vi "DecodeTopicSubscribeReply.vi"(3 "Topic Reply":string="POST / HTTP/1.1\r\nUser-Agent: XMLRPC++ 0.7\r\nHost: 192.168.1.111:5000\r\nContent-Type: text/xml\r\nContent-length: 330\r\n\r\n<?xml version=\"1.0\"?>\r\n<methodCall><methodName>requestTopic</methodName>\r\n<params><param><value>/realtime_loop</value></param><param><value>/robot/head/command_head_nod</value></param><param><value><array><data><value><array><data><value>TCPROS</value></data></array></value></data></array></value></param></params></methodCall>\r\n") -> (0 "error out":errorcluster, 1 "Reply":T1(array[cluster]))   [LabVIEW 2012]
panel:
  in  "error in (no error)":errorcluster
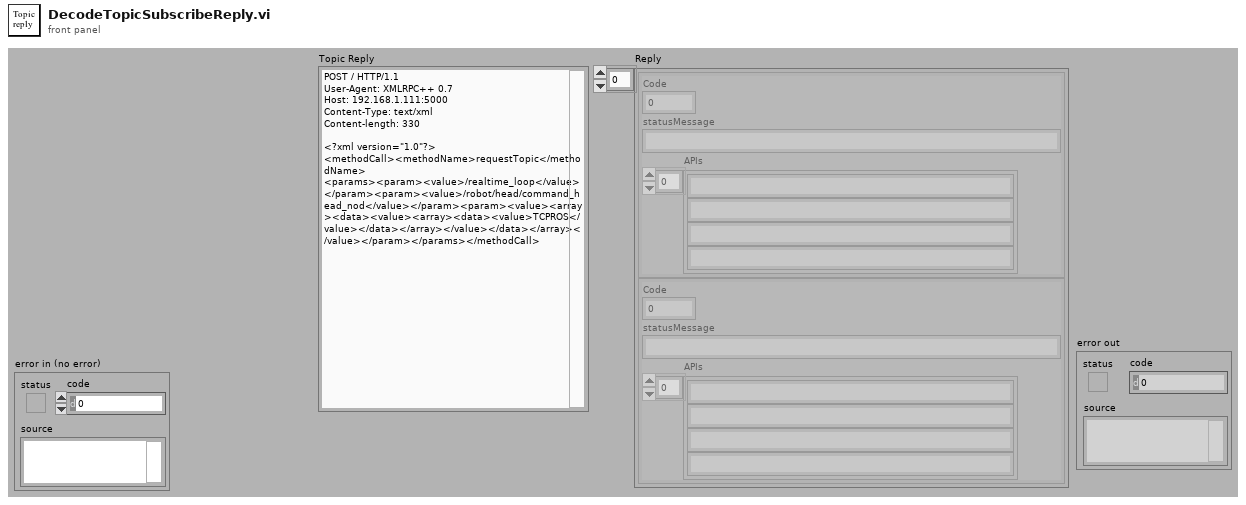
[diagram p1: front panel]
types:
  T1 = cluster{"Code":i8, "statusMessage":string, "APIs":string[]}[]
  T2 = cluster{"Code":i8, "statusMessage":string, "APIs":string[]}
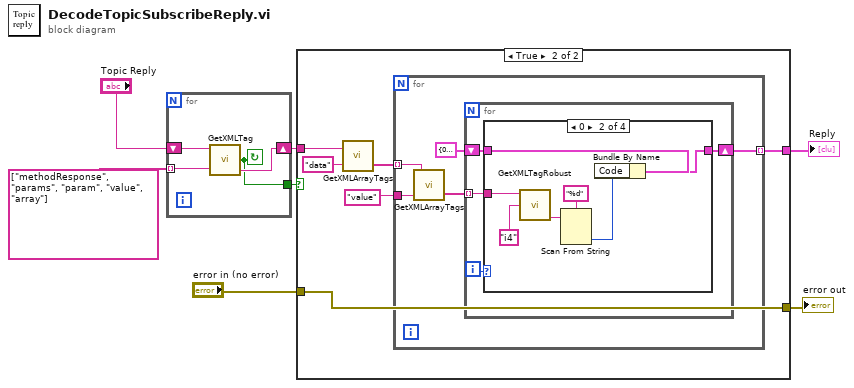
[diagram p0: block diagram]
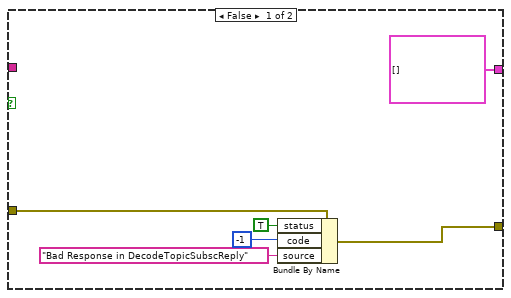
[diagram p2: hidden frame]
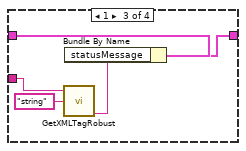
[diagram p4: hidden frame]
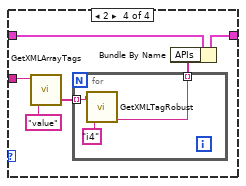
[diagram p5: hidden frame]
diagram:
  n1 = for {
    tunnel: string[] ["methodResponse", "params", "param", "value", "array"] -> [w11] mode=indexing
    shift-right: [w9] -> w6
    shift-left: "Topic Reply" -> [w10]
    tunnel: [w8] -> w4
    stop <- w8 continue-if-true
    n2 = call <userlib>:"GetXMLTag.vi"("Tag"=w11, "String"=w10) -> ("Value"=w9:string, "Exists?"=w8:bool)  [unwired: 1 out]
  }
  n3 = case shown="True" w4 {
    tunnel: w6 -> [_ w20]
    tunnel: [T1 [] w19] -> w5
    tunnel: "error in (no error)" -> [w16 w18]
    tunnel: [w15 w18] -> w2
    frame False {
      n4 = Bundle By Name(cluster=w16, "status"=TRUE, "code"=-1, "source"="Bad Response in DecodeTopicSubscReply") -> (w15:errorcluster)
    }
    frame True {
      n5 = call <userlib>:"GetXMLArrayTags.vi"("ArrayTag"="data", "String"=w20) -> ("Array"=w22:string[])  [unwired: 1 out]
      n6 = for {
        tunnel: w22 -> [w28] mode=indexing
        tunnel: "value" -> [w27]
        tunnel: [w24] -> w19 mode=indexing
        n7 = call <userlib>:"GetXMLArrayTags.vi"("ArrayTag"=w27, "String"=w28) -> ("Array"=w26:string[])  [unwired: 1 out]
        n8 = for {
          tunnel: w26 -> [w32] mode=indexing
          shift-right: [w29] -> w24
          shift-left: T2 {"Code"=0, "statusMessage"="", "APIs"=[]} ("Parameters") -> [w30]
          i -> [w31]
          n9 = case shown="0" w31 {
            tunnel: w32 -> [_ w35 w43 w49]
            tunnel: w30 -> [w33 w38 w45 w51]
            tunnel: [w33 w36 w44 w50] -> w29
            frame Default {
            }
            frame 0 {
              n10 = call <userlib>:"GetXMLTagRobust.vi"("Tag"="i4", "String"=w35) -> ("value"=w34:string)  [unwired: 1 in, 3 out]
              n11 = Scan From String(format string="%d", input string=w34) -> (output 1=w37:i32)  [unwired: 3 in, 3 out]
              n12 = Bundle By Name(cluster=w38, "Code"=w37) -> (w36:T2)
            }
            frame 1 {
              n13 = call <userlib>:"GetXMLTagRobust.vi"("Tag"="string", "String"=w43) -> ("value"=w41:string)  [unwired: 1 in, 3 out]
              n14 = Bundle By Name(cluster=w45, "statusMessage"=w41) -> (w44:T2)
            }
            frame 2 {
              n15 = call <userlib>:"GetXMLArrayTags.vi"("ArrayTag"="value", "String"=w49) -> ("Array"=w47:string[])  [unwired: 1 out]
              n16 = for {
                tunnel: w47 -> [w54] mode=indexing
                tunnel: [w52] -> w46 mode=indexing
                n17 = call <userlib>:"GetXMLTagRobust.vi"("Tag"="i4", "String"=w54) -> ("value"=w52:string)  [unwired: 1 in, 3 out]
              }
              n18 = Bundle By Name(cluster=w51, "APIs"=w46) -> (w50:T2)
            }
          }
        }
      }
    }
  }
  "Reply" <- w5
  "error out" <- w2
